vi "DeleteDataM.vi"(8 "error in (no error)":errorcluster caption="entrée d'erreur (pas d'erreur)", 10 "CurveNumbers":i32[](array[numeric]), 11 "Interface en entrée":refnum<class "Interface.lvclass"> caption="DNL_LabVIEW Object in") -> (0 "error out":errorcluster caption="sortie d'erreur", 3 "Interface en sortie":refnum<class "Interface.lvclass"> caption="DNL_LabVIEW Object out")   [LabVIEW 2019, in "Interface.lvclass"]
uses:
  Interface.lvclass
  Interface.lvclass/Interface.ctl
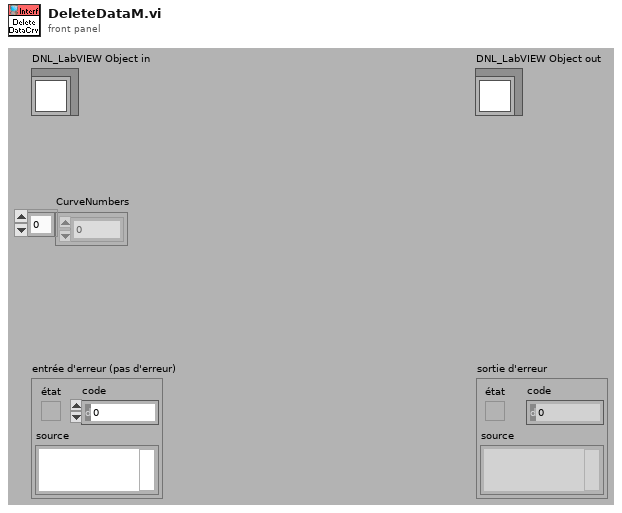
[diagram p1: front panel]
types:
  T1 = typedef "Interface.lvclass/CurveSetup.ctl" = cluster{"CurveName":string, "YParam":string, "XParam":string, "ZParam ":string, "GroupName":string, "LinWdth":u8, "PntCol":u32, "LinCol":u32, "LablFor":u8, "XScale":u32, "YScale":u32, "Interpol":u8, "DisplayName":string, "FillType":i16, "LineStyle":u8, "PntStyle":u8, "BarTyp":u8, "GraphIndex":i32, "Visible":bool, "XScaleName":string, "YScaleName":string, "XYGraph_Ref":refnum<vi>, "Data Only":bool, "DataQ Ref":refnum<queue>, "XParQ Ref":refnum<queue>, "XParamInd":i32, "ScanInd":i32, "File Path":path}
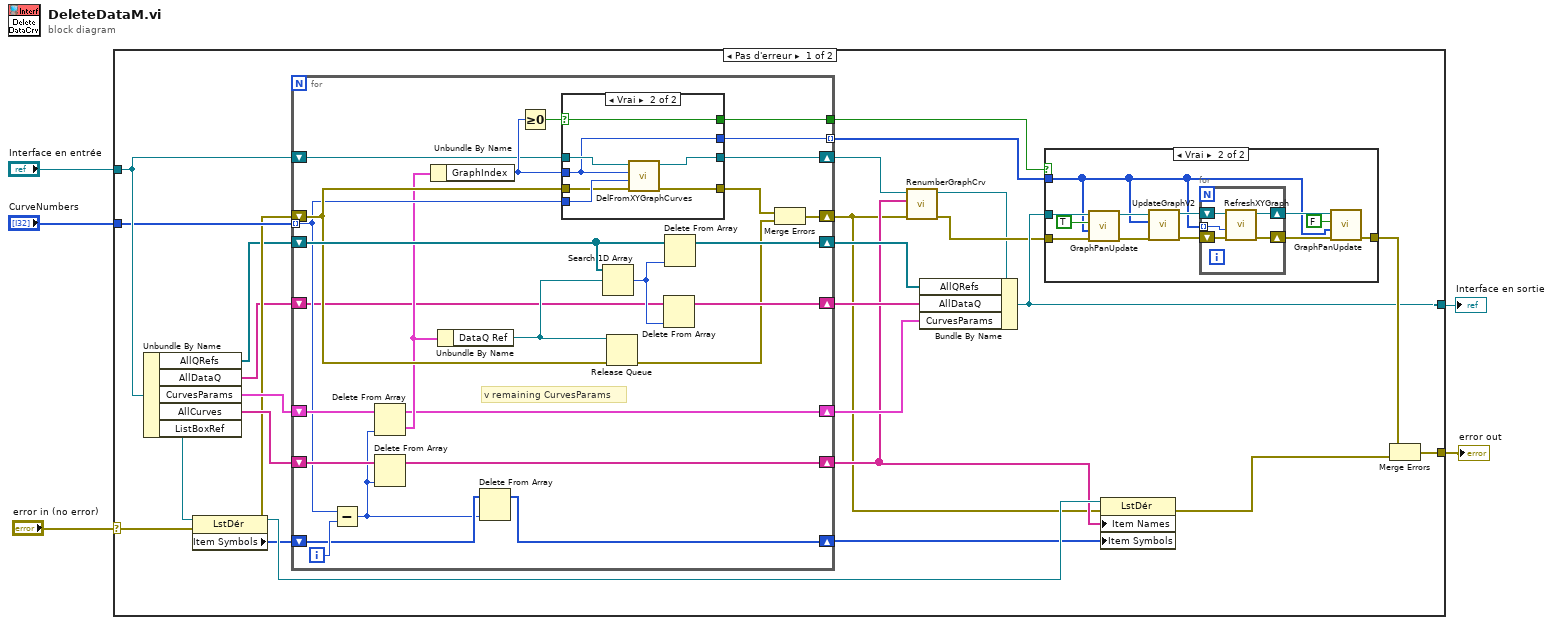
[diagram p0: block diagram]
diagram:
  n1 = case shown="Pas d'erreur" "error in (no error)" {
    selector: "error in (no error)" -> [w27 w88]
    tunnel: [w24 w88] -> w4
    tunnel: [w16 w87] -> w2
    tunnel: "Interface en entrée" -> [w31 w87]
    tunnel: "CurveNumbers" -> [w28 _]
    frame No Error {
      n2 = Unbundle By Name(w31) -> ("AllQRefs"=w12:refnum<queue>[], "AllDataQ"=w13:string[], "CurvesParams"=w29:T1[], "AllCurves"=w30:string[], "ListBoxRef"=w22:refnum<vi>)
      n3 = property class="LstDér"(reference=w22, error in=w27) -> (reference out=w21:refnum<vi>, error out=w17:errorcluster, "Item Symbols"=w18:i32[])
      n4 = for {
        tunnel: w28 -> [w45] mode=indexing
        tunnel: [w49] -> w26
        tunnel: [w48] -> w25 mode=indexing
        shift-right: [w35] -> w7
        shift-left: w31 -> [w56]
        shift-right: [w33] -> w6
        shift-left: w17 -> [w51]
        shift-right: [w44] -> w20
        shift-left: w18 -> [w43]
        shift-right: [w42] -> w10
        shift-left: w30 -> [w55]
        shift-right: [w38] -> w14
        shift-left: w29 -> [w54]
        shift-right: [w39] -> w15
        shift-left: w13 -> [w37]
        shift-right: [w36] -> w11
        shift-left: w12 -> [w53]
        i -> [w46]
        # "v remaining CurvesParams"
        n5 = Subtract(x=w45, y=w46) -> (x-y=w41:i32)
        n6 = Delete From Array(array=w54, index=w41) -> (deleted portion=w40:T1, array with subset deleted=w38:T1[])  [unwired: 1 in]
        n7 = Delete From Array(array=w55, index=w41) -> (array with subset deleted=w42:string[])  [unwired: 1 in, 1 out]
        n8 = Unbundle By Name(w40) -> ("GraphIndex"=w57:i32)
        n9 = Unbundle By Name(w40) -> ("DataQ Ref"=w52:refnum<queue>)
        n10 = Delete From Array(array=w43, index=w41) -> (array with subset deleted=w44:i32[])  [unwired: 1 in, 1 out]
        n11 = Greater Or Equal To 0?(x=w57) -> (x >= 0?=w50:bool)
        n12 = case shown="Vrai" w50 {
          selector: w50 -> [w60 w64]
          tunnel: w45 -> [_ w67]
          tunnel: w57 -> [w59 w65]
          tunnel: w56 -> [w58 w68]
          tunnel: w51 -> [w61 w66]
          tunnel: [w61 w62] -> w32
          tunnel: [w59 w65] -> w48
          tunnel: [w60 w64] -> w49
          tunnel: [w58 w63] -> w35
          frame False {
            # "curves was not graphed"
          }
          frame True {
            n13 = call "DelFromXYGraphCurves.vi"("error in (no error)"=w66, "CurvIndex"=w67, "GraphIndex"=w65, "Interface en entrée"=w68) -> ("error out"=w62:errorcluster, "Interface en sortie"=w63:refnum<class "Interface.lvclass">)  [unwired: 6 in]
          }
        }
        n14 = Search 1D Array(1D array=w53, element=w52) -> (index of element=w47:i32)  [unwired: 1 in]
        n15 = Release Queue(queue=w52, error in (no error)=w51) -> (error out=w34:errorcluster)  [unwired: 1 in, 2 out]
        n16 = Delete From Array(array=w37, index=w47) -> (array with subset deleted=w39:string[])  [unwired: 1 in, 1 out]
        n17 = Delete From Array(array=w53, index=w47) -> (array with subset deleted=w36:refnum<queue>[])  [unwired: 1 in, 1 out]
        n18 = Merge Errors(w32, w34) -> (w33:errorcluster)
      }
      n19 = call "RenumberGraphCrv.vi"("error in (no error)"=w6, "AllCurves"=w10, "Interface en entrée"=w7) -> ("error out"=w9:errorcluster, "Interface en sortie"=w8:refnum<class "Interface.lvclass">)  [unwired: 7 in]
      n20 = Bundle By Name(cluster=w8, "AllQRefs"=w11, "AllDataQ"=w15, "CurvesParams"=w14) -> (w16:refnum<class "Interface.lvclass">)
      n21 = case shown="Vrai" w26 {
        tunnel: w16 -> [_ w73]
        tunnel: w25 -> [_ w70]
        tunnel: w9 -> [w69 w72]
        tunnel: [w69 w71] -> w23
        frame False {
        }
        frame True {
          n22 = call "GraphPanUpdate.vi"("error in (no error)"=w72, "GraphInd"=w70, "DeferUpdate"=TRUE, "Interface en entrée"=w73) -> ("error out"=w81:errorcluster, "Interface en sortie"=w80:refnum<class "Interface.lvclass">)  [unwired: 6 in]
          n23 = call "UpdateGraphV2.vi"("error in (no error)"=w81, "GraphIndexArr"=w70, "Interface en entrée"=w80) -> ("error out"=w76:errorcluster, "Interface en sortie"=w78:refnum<class "Interface.lvclass">)  [unwired: 7 in]
          n24 = for {
            shift-right: [w86] -> w79
            shift-left: w78 -> [w85]
            shift-right: [w84] -> w77
            shift-left: w76 -> [w83]
            tunnel: w70 -> [w82] mode=indexing
            n25 = call "RefreshXYGraph.vi"("error in (no error)"=w83, "Graph Index"=w82, "Interface en entrée"=w85) -> ("error out"=w84:errorcluster, "Interface en sortie"=w86:refnum<class "Interface.lvclass">)  [unwired: 6 in, 1 out]
          }
          n26 = call "GraphPanUpdate.vi"("error in (no error)"=w77, "GraphInd"=w70, "DeferUpdate"=FALSE, "Interface en entrée"=w79) -> ("error out"=w71:errorcluster)  [unwired: 6 in, 1 out]
        }
      }
      n27 = property class="LstDér"(reference=w21, error in=w6, "Item Names"=w10, "Item Symbols"=w20) -> (error out=w19:errorcluster)  [unwired: 1 out]
      n28 = Merge Errors(w23, w19) -> (w24:errorcluster)
    }
    frame Error {
    }
  }
  "error out" <- w4
  "Interface en sortie" <- w2
